vi "Write cfg file folder.vi"(8 "error in (no error)":errorcluster, 10 "cfg file folder":path, 11 "[V] Sys Cfg Base in":refnum<class "[V] Sys Cfg Base.lvclass">) -> (0 "error out":errorcluster, 3 "[V] Sys Cfg Base out":refnum<class "[V] Sys Cfg Base.lvclass">)   [LabVIEW 2023, in "[V] Sys Cfg Base.lvlib" / "[V] Sys Cfg Base.lvclass"]
uses:
  [V] Sys Cfg Base.lvclass
  [V] Sys Cfg Base.lvclass/[V] Sys Cfg Base.ctl
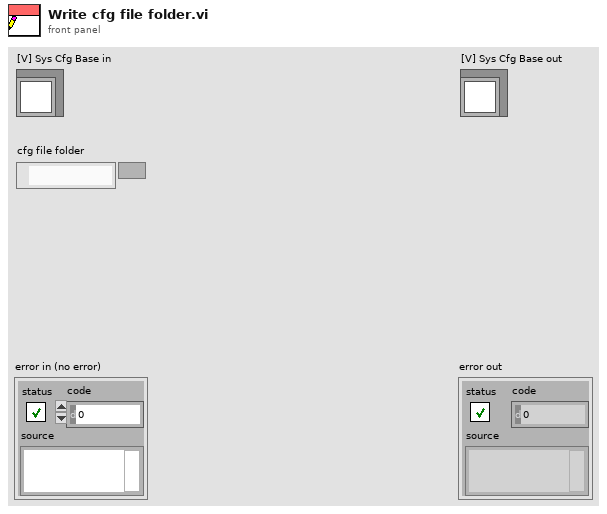
[diagram p1: front panel]
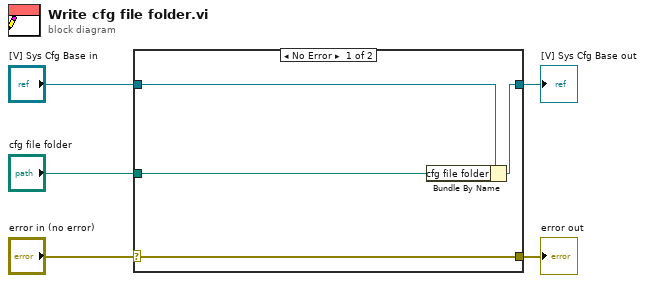
[diagram p0: block diagram]
diagram:
  n1 = case shown="No Error" "error in (no error)" {
    selector: "error in (no error)" -> [w9 w10]
    tunnel: [w9 w10] -> w4
    tunnel: [w7 w11] -> w2
    tunnel: "[V] Sys Cfg Base in" -> [w8 w11]
    tunnel: "cfg file folder" -> [w6 _]
    frame No Error {
      n2 = Bundle By Name(cluster=w8, "cfg file folder"=w6) -> (w7:refnum<class "[V] Sys Cfg Base.lvclass">)
    }
    frame Error {
    }
  }
  "error out" <- w4
  "[V] Sys Cfg Base out" <- w2
